vi "Client Processing Loop Sandbox.vi"() -> ()   [LabVIEW 2014]
uses:
  System/Classes/Topic_class/Topic.lvclass
panel:
  in  "error in":errorcluster
  in  "Client Name":string
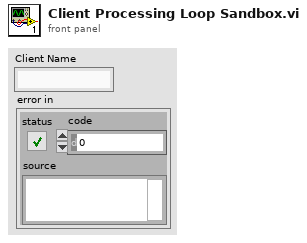
[diagram p1: front panel]
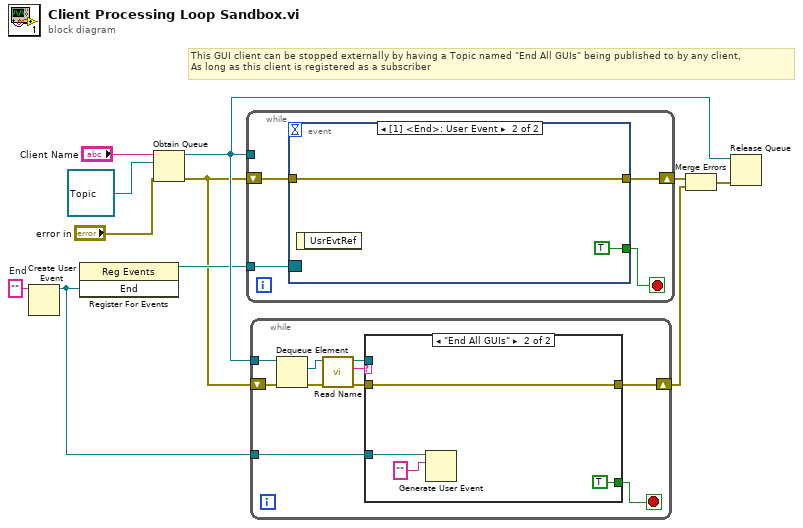
[diagram p0: block diagram]
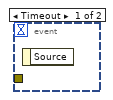
[diagram p3: hidden frame]
diagram:
  w7 = ""  # End
  # "This GUI client can be stopped externally by having a Topic named \"End All GUIs\" being published to by any client,\nAs long as this client is registered as a subscriber"
  n1 = Create User Event(user event datatype=w7) -> (user event=w5:refnum<user-event>)  [unwired: 1 in, 1 out]
  n2 = register-events(w5) -> (reference out=w6:refnum<event-registration>)  [unwired: 2 in, 1 out]
  n3 = Obtain Queue(name (unnamed)="Client Name", element data type=refnum<class "Topic.lvclass"> refnum ("Topic.lvclass"), error in (no error)="error in") -> (queue out=w9:refnum<queue>, error out=w4:errorcluster)  [unwired: 2 in, 1 out]
  n4 = while {
    tunnel: w9 -> [_]
    tunnel: w6 -> [w15]
    shift-right: [w12] -> w3
    shift-left: w4 -> [w13]
    stop <- w14 stop-if-true
    n5 = event shown="[1] <End>: User Event" {
      selector: w15 -> [_ _]
      dyn-events: _ -> [_ _]
      timeout: _ -> [_ _]
      tunnel: [_ TRUE] -> w14
      tunnel: w13 -> [_ w16]
      tunnel: [_ w16] -> w12
      event Timeout {
        n6 = event-data() -> ()  [unwired: 1 in, 1 out]
      }
      event User Event {
        n7 = event-data() -> ()  [unwired: 1 in, 1 out]
      }
    }
  }
  n8 = while {
    tunnel: w9 -> [w25]
    tunnel: w5 -> [w20]
    shift-right: [w18] -> w2
    shift-left: w4 -> [w22]
    stop <- w21 stop-if-true
    n9 = Dequeue Element(queue=w25, error in (no error)=w22) -> (element=w24:refnum<class "Topic.lvclass">, error out=w23:errorcluster)  [unwired: 1 in, 2 out]
    n10 = call-dynamic "Read Name.vi"("error in"=w23, "Topic in"=w24) -> ("error out"=w19:errorcluster, "Name"=w27:string, "Topic out"=w26:refnum<class "Topic.lvclass">)  [unwired: 7 in]
    n11 = case shown="\"End All GUIs\"" w27 {
      tunnel: w26 -> [_ _]
      tunnel: [_ TRUE] -> w21
      tunnel: w20 -> [_ w31]
      tunnel: w19 -> [w28 w29]
      tunnel: [w28 w29] -> w18
      frame Default {
      }
      frame "End All GUIs" {
        n12 = Generate User Event(user event=w31, event data cluster="" ("event data")) -> ()  [unwired: 2 in, 2 out]
      }
    }
  }
  n13 = Merge Errors(w3, w2) -> (w1:errorcluster)
  n14 = Release Queue(queue=w9, error in (no error)=w1) -> ()  [unwired: 1 in, 3 out]
